vi "Timeout.vi"(8 "error in (no error)":errorcluster, 11 "Freezer in":refnum<class "Freezer.lvclass">=refnum) -> (0 "error out":errorcluster, 3 "Freezer out":refnum<class "Freezer.lvclass">)   [LabVIEW 2015, in "Freezer.lvclass"]
uses:
  Freezer.lvclass
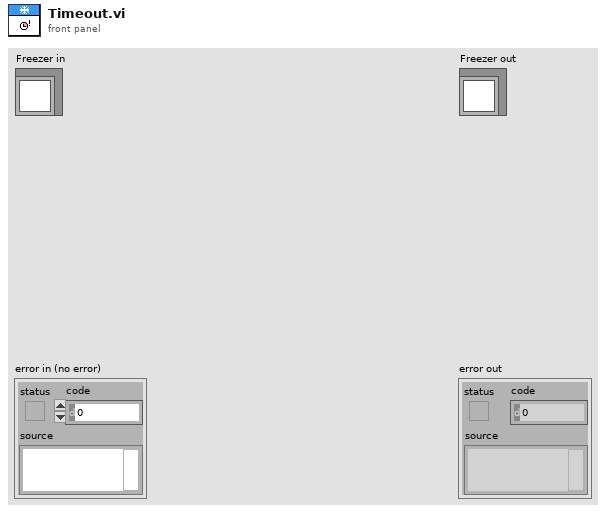
[diagram p1: front panel]
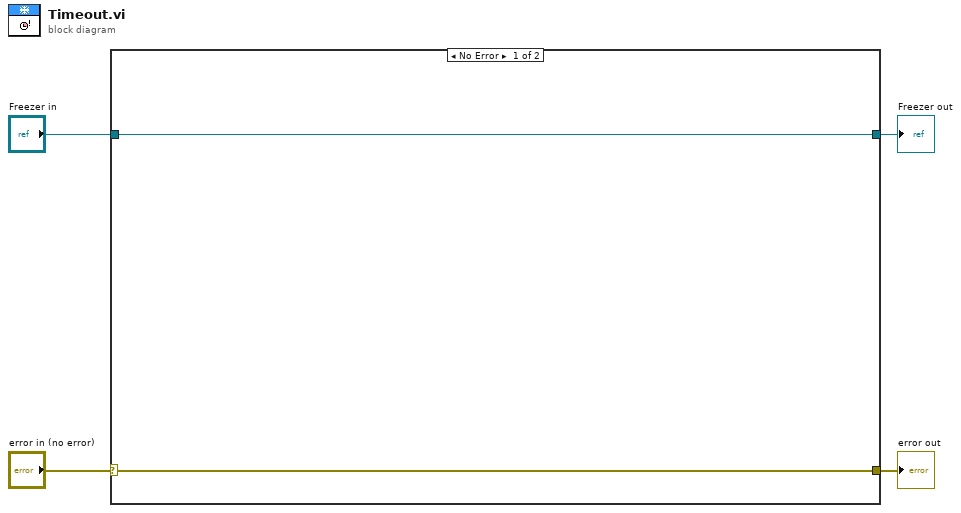
[diagram p0: block diagram]
diagram:
  n1 = case shown="No Error" "error in (no error)" {
    selector: "error in (no error)" -> [w5 w8]
    tunnel: [w5 w8] -> w3
    tunnel: [w6 w7] -> w2
    tunnel: "Freezer in" -> [w6 w7]
    frame No Error {
    }
    frame Error {
    }
  }
  "error out" <- w3
  "Freezer out" <- w2
